vi "json Parse Path Array - array path.vi"(8 "error in (no error)":errorcluster, 9 "default":path[](array[path]), 10 "path":string[](array[string]), 11 "JSON Document in":refnum<class "JSON Document.lvclass">) -> (0 "error out":errorcluster, 1 "defaulted?":bool, 2 "value":path[](array[path]), 3 "JSON Document out":refnum<class "JSON Document.lvclass">, 4 "elements defaulted?":bool[](array[boolean]))   [LabVIEW 2015, in "JSON Document.lvclass"]
uses:
  JSON Document.lvclass
  json Parse Path Array - string path.vi
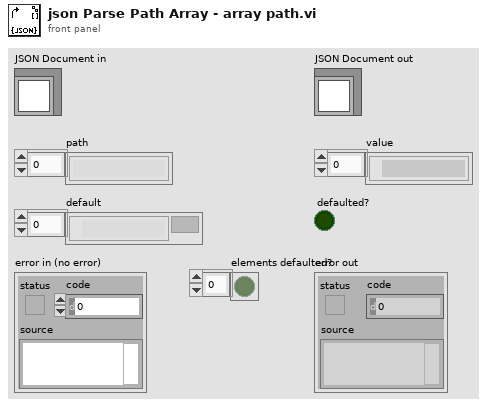
[diagram p1: front panel]
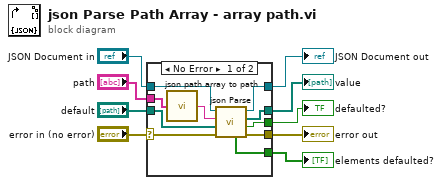
[diagram p0: block diagram]
diagram:
  n1 = case shown="No Error" "error in (no error)" {
    selector: "error in (no error)" -> [w16 w22]
    tunnel: [w10 w22] -> w8
    tunnel: [w14 w21] -> w6
    tunnel: "JSON Document in" -> [w15 w21]
    tunnel: "default" -> [w17 w20]
    tunnel: "path" -> [w19 _]
    tunnel: [w12 w20] -> w3
    tunnel: [w13 _] -> w2
    tunnel: [w11 _] -> w1
    frame No Error {
      n2 = call "json path array to path.vi"("path"=w19) -> ("String"=w18:string)
      n3 = call-poly "json Parse.vi"("error in (no error)"=w16, "default"=w17, "path"=w18, "JSON Document in"=w15) -> ("error out"=w10:errorcluster, "defaulted?"=w13:bool, "value"=w12:path[], "JSON Document out"=w14:refnum<class "JSON Document.lvclass">, "elements defaulted?"=w11:bool[])  [unwired: 3 in]
    }
    frame Error {
    }
  }
  "error out" <- w8
  "JSON Document out" <- w6
  "value" <- w3
  "defaulted?" <- w2
  "elements defaulted?" <- w1
